vi "Do.vi"(8 "error in (no error)":errorcluster, 10 "Actor in":refnum<class "Actor.lvclass">, 11 "Instrument Msg":refnum<class "Instrument Handler Response Msg.lvclass">) -> (0 "error out":errorcluster, 2 "Actor out":refnum<class "Actor.lvclass">)   [LabVIEW 2020, in "Instrument Handler.lvlib" / "Instrument Handler Response Msg.lvclass"]
doc: "This implementation will forward the message to the Instrument Handler where it will execute."
uses:
  Instrument Handler Response Msg.lvclass
  C:/Current projects/WS/PPL/HDH.Actor Framework.Core.Publisher.lvlibp/Messages/Response Msg/Response Msg.lvclass
  PPL/HDH.Actor Framework.Core.Actor.lvlibp/1abvi3w/vi.lib/ActorFramework/Actor/Actor.lvclass
  Instrument Handler/Instrument Handler.lvclass
  Instrument Handler Response Msg.lvclass/Instrument Handler Response Msg.ctl
  PPL/HDH.Actor Framework.Core.Publisher.lvlibp/Publisher Messages/Targetted Msg/Targetted Msg.lvclass
  C:/Current projects/WS/PPL/HDH.Actor Framework.Core.Publisher.lvlibp/Publisher Messages/Sender Msg/Sender Msg.lvclass
  PPL/HDH.Actor Framework.Core.Publisher.lvlibp/Messages/Response Msg/Response Msg.lvclass
  C:/Current projects/WS/PPL/HDH.Actor Framework.Core.Actor.lvlibp/1abvi3w/vi.lib/ActorFramework/Actor/Actor.lvclass
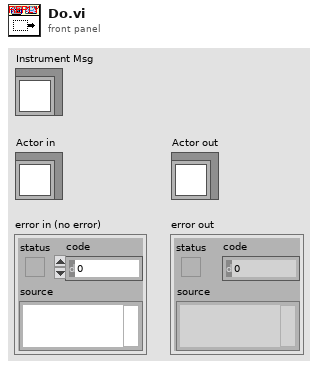
[diagram p1: front panel]
types:
  T1 = typedef "HDH.Actor Framework.Core.Publisher.lvlibp/Ctl_SendFunction.ctl" = enum16{"Send and Forget", "Request Reply", "Await Reply"}
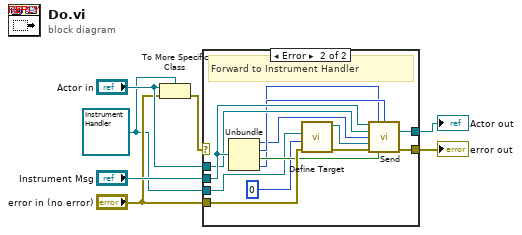
[diagram p0: block diagram]
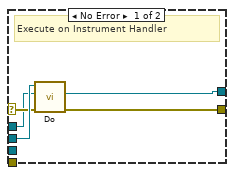
[diagram p2: hidden frame]
diagram:
  w1 = refnum<class "Instrument Handler.lvclass"> refnum ("Instrument Handler.lvlib:Instrument Handler.lvclass")
  n1 = To More Specific Class(target class=w1, reference="Actor in", error in="error in (no error)") -> (error out=w4:errorcluster)  [unwired: 1 out]
  n2 = case shown="Error" w4 {
    selector: w4 -> [w9 _]
    tunnel: [w12 w23] -> w7
    tunnel: [w11 w24] -> w6
    tunnel: "Instrument Msg" -> [w10 w22]
    tunnel: "Actor in" -> [w8 w21]
    tunnel: "error in (no error)" -> [_ w25]
    tunnel: w1 -> [_ w14]
    frame No Error {
      # "Execute on Instrument Handler"
      n3 = call-parent "Do.vi"("error in (no error)"=w9, "Actor in"=w8, "Response Msg"=w10) -> ("error out"=w12:errorcluster, "Actor out"=w11:refnum<class "Actor.lvclass">)  [unwired: 7 in]
    }
    frame Error {
      # "Forward to Instrument Handler"
      n4 = Unbundle(w22) -> (w17:T1, w20:i32, w19:bool, w13:u16)
      n5 = call "Define Target.vi"("error in (no error)"=w25, "Target Actor index(-1, all)"=0, "Target Actor"=w14) -> ("error out"=w16:errorcluster, "Targetted Msg out"=w18:refnum<class "Targetted Msg.lvclass">)  [unwired: 7 in]
      n6 = call "Send.vi"("Response Msg in"=w22, "Message Priority (Normal)"=w13, "Timeout if waiting(-1ms)"=w20, "Actor in"=w21, "Send Function"=w17, "Sender (publish)"=w18, "error in (no error)"=w16, "Publish Data?(F)"=w19) -> ("Actor out"=w24:refnum<class "Actor.lvclass">, "error out"=w23:errorcluster)  [unwired: 3 in, 3 out]
    }
  }
  "error out" <- w7
  "Actor out" <- w6
